vi "Default Setup.vi"(8 "error in (no error)":errorcluster, 11 "VISA resource name":refnum<visa-resource-name>) -> (0 "error out":errorcluster, 3 "VISA resource name out":refnum<visa-resource-name>)   [LabVIEW 2019, in "DS360.lvlib"]
uses:
  DS360.lvlib
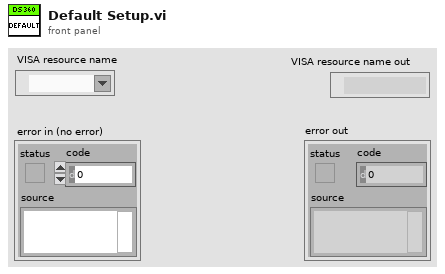
[diagram p1: front panel]
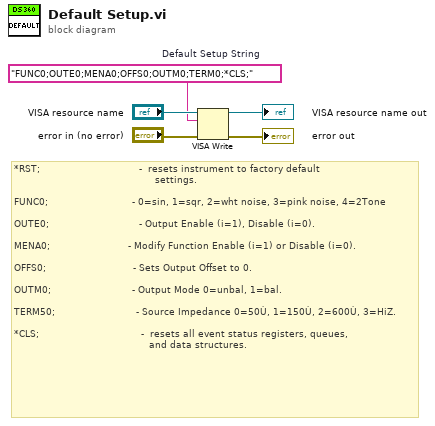
[diagram p0: block diagram]
diagram:
  w1 = "FUNC0;OUTE0;MENA0;OFFS0;OUTM0;TERM0;*CLS;"  # Default Setup String
  # "*RST;                                 -  resets instrument to factory default \n                                               settings.\n\nFUNC0;                            - 0=sin, 1=sqr, 2=wht noise, 3=pink noise, 4=2Tone \n\nOUTE0;                              - Output Enable (i=1), Disable (i=0).\n\nMENA0;                          - Modify Function Enable (i=1) or Disable (i=0).\n\nOFFS0;                             - Sets Output Offset to 0.\n\nOUTM0;                           - Output Mode 0=unbal, 1=bal.\n\nTERM50;                           - Source Impedance 0=50Ù, 1=150Ù, 2=600Ù, 3=HiZ.\n\n*CLS;                                  -  resets all event status registers, queues,\n                                             and data structures."
  n1 = VISA Write(VISA resource name="VISA resource name", write buffer=w1, error in (no error)="error in (no error)") -> (VISA resource name out=→"VISA resource name out":refnum<visa-resource-name>, error out=→"error out":errorcluster)  [unwired: 1 out]
